vi "Write Config.vi"(8 "error in (no error)":errorcluster, 9 "Re-Init?":bool, 10 "ICM File In":path, 11 "Scaling in":refnum<class "Scaling.lvclass">) -> (0 "error out":errorcluster, 3 "Scaling out":refnum<class "Scaling.lvclass">)   [LabVIEW 2018, in "Scaling.lvclass"]
doc: "Scaling.lvclass:Write Config.vi\n\nThis is the template for the Write Config VI for the Scaling class.\n\nInstrument Communication Module Version 1.0\nSeptember, 2017 Original Code Consulting David Thomson\n www.originalcode.com"
uses:
  Scaling.lvclass
  Scaling.lvclass/Scaling.ctl
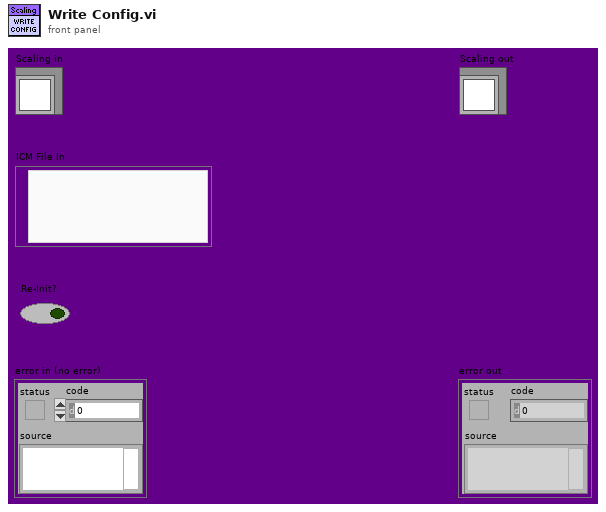
[diagram p1: front panel]
types:
  T1 = typedef "Scaling Def.ctl" = cluster{"Channel":string, "Scaling":string, "Instance":string}
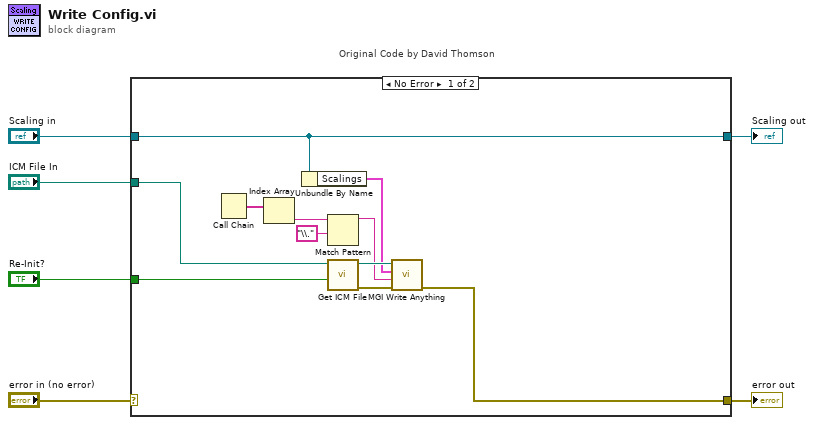
[diagram p0: block diagram]
diagram:
  n1 = case "Original Code by David Thomson" shown="No Error" "error in (no error)" {
    selector: "error in (no error)" -> [_ w19]
    tunnel: [w7 w19] -> w5
    tunnel: [w10 w18] -> w3
    tunnel: "Scaling in" -> [w10 w18]
    tunnel: "ICM File In" -> [w9 _]
    tunnel: "Re-Init?" -> [w8 _]
    frame No Error {
      n2 = Call Chain() -> (call chain=w16:string[])
      n3 = Index Array(array=w16) -> (element=w15:string)  [unwired: 1 in]
      n4 = Unbundle By Name(w10) -> ("Scalings"=w11:T1[])
      n5 = Match Pattern(string=w15, regular expression="\\.") -> (before substring=w12:string)  [unwired: 1 in, 3 out]
      n6 = call "Get ICM File.vi"("Re-Init?"=w8, "ICM File In"=w9) -> ("error out"=w14:errorcluster, "ICM File"=w13:path)  [unwired: 8 in]
      n7 = call "MGI Write Anything.vi"("Error In"=w14, "Section Name (Name of \"Anything\")"=w12, "Anything"=w11, "Path (dialog)"=w13) -> ("Error Out"=w7:errorcluster)  [unwired: 5 in, 2 out]
    }
    frame Error {
    }
  }
  "error out" <- w5
  "Scaling out" <- w3
